vi "test Should Return Call Parameters.vi"(8 "error in (no error)":errorcluster, 11 "TestCase in":refnum<class "Store and Return Parameters.lvclass">) -> (0 "error out":errorcluster, 3 "TestCase out":refnum<class "Store and Return Parameters.lvclass">)   [LabVIEW 2013, in "Store and Return Parameters.lvclass"]
uses:
  Store and Return Parameters.lvclass
  Core Classes/LabSpy/LabSpy.lvclass
  <vilib>/addons/_JKI Toolkits/VI Tester/TestCase.llb/TestCase.lvclass
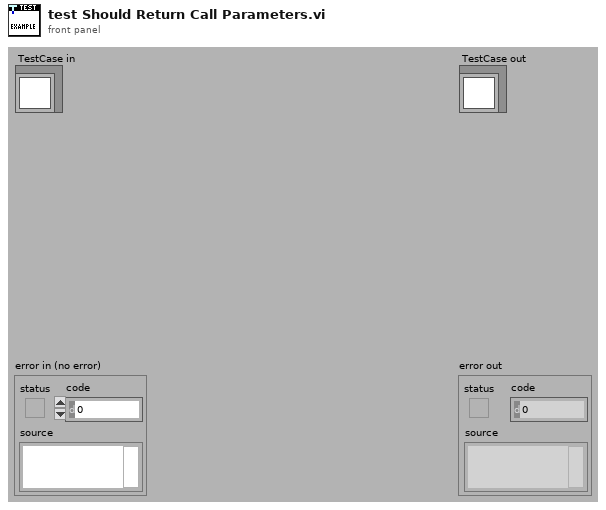
[diagram p1: front panel]
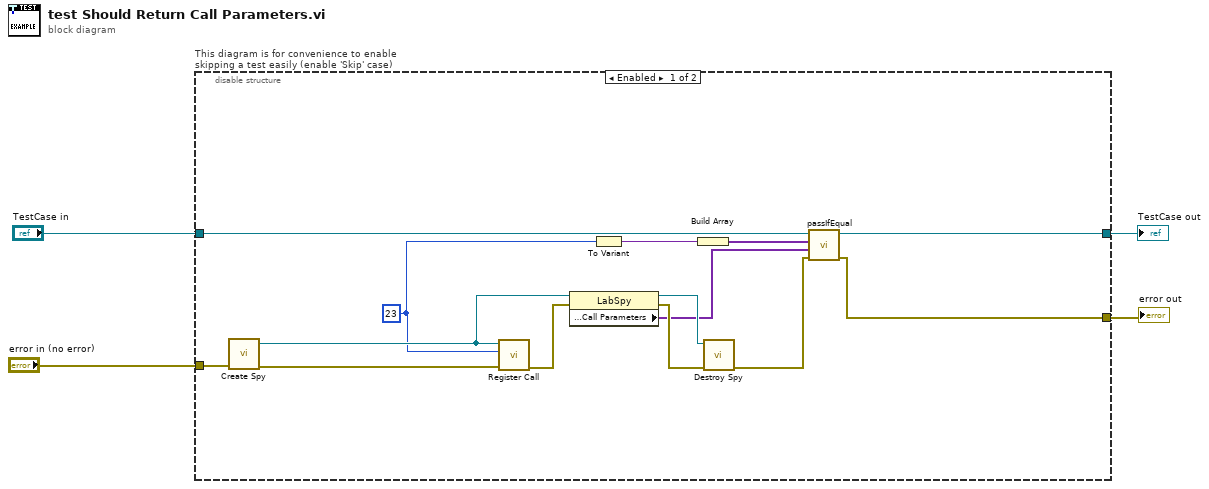
[diagram p0: block diagram]
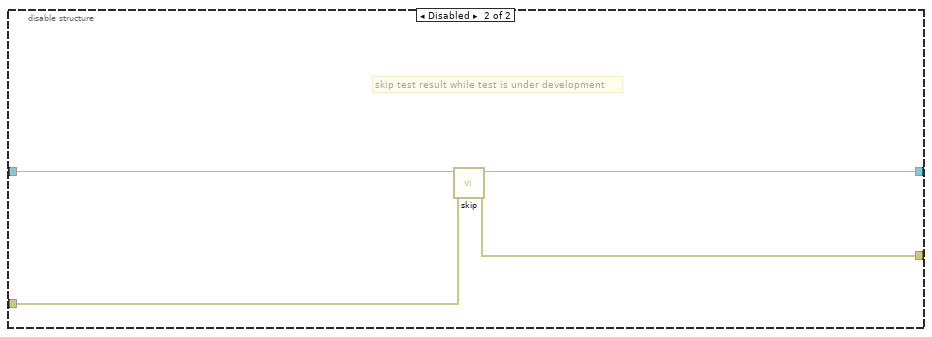
[diagram p2: hidden frame]
diagram:
  n1 = disable-structure "This diagram is for convenience to enable skipping a test easily (enable 'Skip' case)" shown="Enabled" {
    disable-tunnel: "TestCase in" -> [w12 w22]
    disable-tunnel: [w11 w20] -> w1
    disable-tunnel: [w10 w21] -> w3
    disable-tunnel: "error in (no error)" -> [w18 w19]
    frame Enabled {
      w7 = 23
      n2 = call "Create Spy.vi"("error in (no error)"=w18) -> ("error out"=w17:errorcluster, "LabSpy Out"=w16:refnum<data-value>)  [unwired: 9 in]
      n3 = call "Register Call.vi"("error in (no error)"=w17, "Parameters"=w7, "LabSpy"=w16) -> ("error out"=w15:errorcluster)  [unwired: 7 in, 1 out]
      n4 = property class="LabSpy"(reference=w16, error in=w15) -> (reference out=w13:refnum<data-value>, error out=w14:errorcluster, "Parameter Readings:Call Parameters"=w8:variant[])
      n5 = To Variant(anything=w7) -> (Variant=w6:variant)
      n6 = Build Array(w6) -> (w5:variant[])
      n7 = call "Destroy Spy.vi"("error in (no error)"=w14, "LabSpy"=w13) -> ("error out"=w9:errorcluster)  [unwired: 9 in]
      n8 = call-dynamic "passIfEqual.vi"("error in (no error)"=w9, "y"=w8, "x"=w5, "TestCase in"=w12) -> ("error out"=w10:errorcluster, "TestCase out"=w11:refnum<class "Store and Return Parameters.lvclass">)  [unwired: 6 in]
    }
    frame Disabled {
      # "skip test result while test is under development"
      n9 = call <vilib>:"skip.vi"("error in (no error)"=w19, "TestCase in"=w22) -> ("error out"=w21:errorcluster, "TestCase out"=w20:refnum<class "Store and Return Parameters.lvclass">)  [unwired: 8 in]
    }
  }
  "error out" <- w3
  "TestCase out" <- w1
